vi "DimIndicators.get_service_info.vi"(0 "controlRef":refnum<vi>, 5 "error in (no error)":errorcluster) -> (14 "controlRef out":refnum<vi>, 15 "serviceName":string, 16 "typeDescriptor":string, 17 "quality":i32, 18 "timeStamp":dbl, 19 "error out":errorcluster)   [LabVIEW 2015, in "DimIndicators.lvlib"]
doc: "Registers a control of one of the types in \"typedefs\" to a DIM service. If no longer used, a registered event should be unregistered using \"release service\"."
uses:
  DimIndicators.lvlib
  DimIndicators.actionType.ctl
  LVDimInterface/LVDimInterface.lvlib
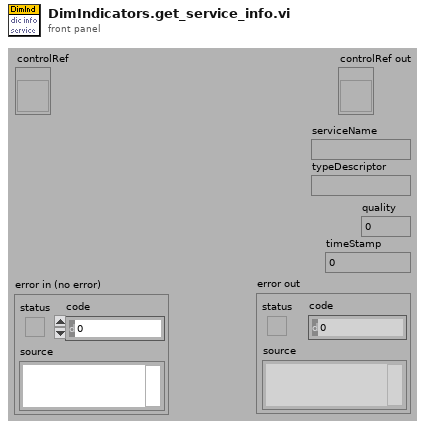
[diagram p1: front panel]
types:
  T1 = typedef "DimIndicators.lvlib/DimIndicators.actionType.ctl" = enum16{"dic_info_service", "dic_release_service", "init", "getControlRef", "getCallbackID", "close"}
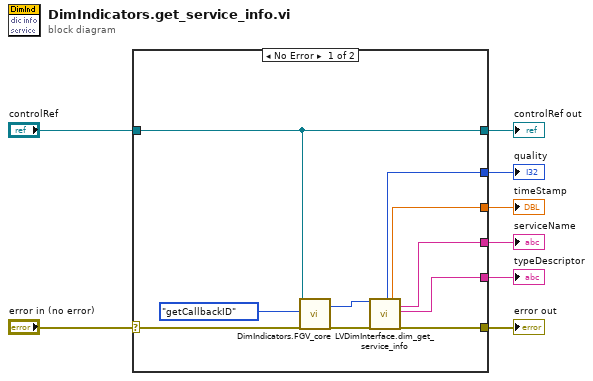
[diagram p0: block diagram]
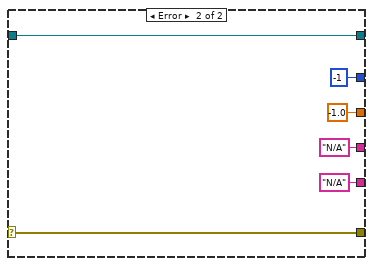
[diagram p2: hidden frame]
diagram:
  n1 = case shown="No Error" "error in (no error)" {
    selector: "error in (no error)" -> [w18 w24]
    tunnel: [w15 w24] -> w7
    tunnel: "controlRef" -> [w14 w23]
    tunnel: [w14 w23] -> w5
    tunnel: [w12 -1 ("quality")] -> w4
    tunnel: [w11 -1.0 ("timeStamp")] -> w3
    tunnel: [w10 "N/A" ("serviceName")] -> w2
    tunnel: [w9 "N/A" ("typeDescriptor")] -> w1
    frame No Error {
      n2 = call "DimIndicators.FGV_core.vi"("controlRef"=w14, "actions"=DimIndicators.actionType."getCallbackID", "error in (no error)"=w18) -> ("callBackID out"=w13:i32, "error out"=w16:errorcluster)  [unwired: 13 in, 2 out]
      n3 = call "LVDimInterface.dim_get_service_info.vi"("callBackID"=w13, "error in (no error)"=w16) -> ("quality"=w12:i32, "timeStamp"=w11:dbl, "serviceName"=w10:string, "typeDescriptor"=w9:string, "error out"=w15:errorcluster)  [unwired: 8 in, 5 out]
    }
    frame Error {
    }
  }
  "error out" <- w7
  "controlRef out" <- w5
  "timeStamp" <- w3
  "quality" <- w4
  "typeDescriptor" <- w1
  "serviceName" <- w2
